vi "CONF config to serial.vi"(7 "Reorder config":bool, 8 "error in (no error)":errorcluster, 10 "AI HW conf array":T1[](array[typedef])) -> (0 "error out":errorcluster, 1 "Config serial out":bool[][](array[boolean]), 2 "Chanel no":i32)   [LabVIEW 2013]
doc: "Konfiguracja kart analogowych\nKonwersja sygnału z wektora konfiguracyjnego\nna ramkę danych dla rejestrów przesuwnych"
uses:
  Kontrolki/KartaDAQ/CONF AI HW config.ctl
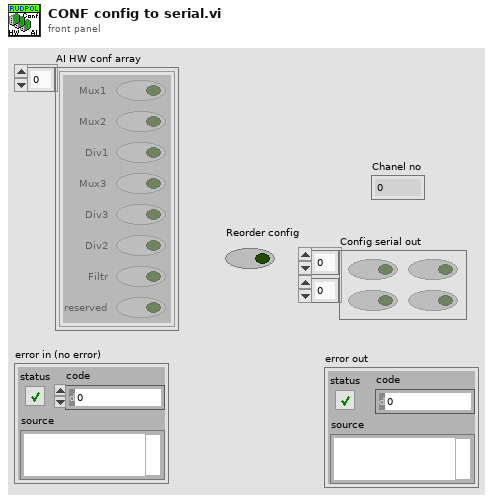
[diagram p1: front panel]
types:
  T1 = typedef "CONF AI HW config.ctl" = cluster{"Mux1":bool, "Mux2":bool, "Div1":bool, "Mux3":bool, "Div3":bool, "Div2":bool, "Filtr":bool, "reserved":bool}
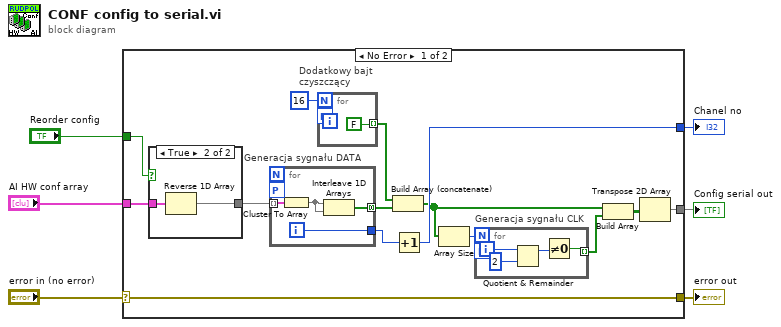
[diagram p0: block diagram]
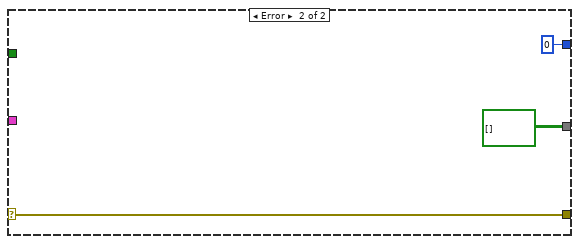
[diagram p3: hidden frame]
diagram:
  n1 = case shown="No Error" "error in (no error)" {
    selector: "error in (no error)" -> [w12 w34]
    tunnel: [w15 bool[][] [] ("element")] -> w3
    tunnel: "AI HW conf array" -> [w13 _]
    tunnel: [w12 w34] -> w6
    tunnel: [w10 0] -> w2
    tunnel: "Reorder config" -> [w7 _]
    frame No Error {
      n2 = case shown="True" w7 {
        tunnel: [w21 w23] -> w14
        tunnel: w13 -> [w21 w22]
        frame False {
        }
        frame True {
          n3 = Reverse 1D Array(array=w22) -> (reversed array=w23:T1[])
        }
      }
      n4 = for "Generacja sygnału DATA" {
        tunnel: w14 -> [w31] mode=indexing
        tunnel: [w32] -> w11
        tunnel: [w29] -> w18 mode=concatenating
        workers-P: _ -> [_]
        i -> [w32]
        n5 = Cluster To Array(cluster=w31) -> (array=w30:bool[])
        n6 = Interleave 1D Arrays(w30, w30) -> (w29:bool[])
      }
      n7 = for "Dodatkowy bajt\nczyszczący" {
        N: 16 -> [_]
        tunnel: [FALSE] -> w19 mode=indexing
        workers-P: _ -> [_]
      }
      n8 = Build Array (concatenate)(w19, w18) -> (w8:bool[])
      n9 = Increment(x=w11) -> (x+1=w10:i32)
      n10 = Array Size(array=w8) -> (size(s)=w17:i32)
      n11 = for "Generacja sygnału CLK" {
        N: w17 -> [_]
        tunnel: [w24] -> w9 mode=indexing
        workers-P: _ -> [_]
        i -> [w27]
        n12 = Quotient & Remainder(x=w27, y=2) -> (x-y*floor(x/y)=w25:i32)  [unwired: 1 out]
        n13 = Not Equal To 0?(x=w25) -> (x != 0?=w24:bool)
      }
      n14 = Build Array(w8, w9) -> (w16:bool[][])
      n15 = Transpose 2D Array(2D array=w16) -> (transposed array=w15:bool[][])
    }
    frame Error {
    }
  }
  "error out" <- w6
  "Config serial out" <- w3
  "Chanel no" <- w2
